vi "TimingDebug.vi"() -> ()   [LabVIEW 2021]
uses:
  <vilib>/DAQmx/read.llb/DAQmx Read (Analog 2D DBL NChan NSamp).vi
  <vilib>/DAQmx/create/channels.llb/DAQmx Create Channel (AI-Voltage-Basic).vi
  <vilib>/DAQmx/configure/timing.llb/DAQmx Timing (Sample Clock).vi
  <vilib>/DAQmx/miscellaneous.llb/DAQmx Fill In Error Info.vi
panel:
  out "data":dbl[][](array[numeric]) format="%0.2f"
  out "Time has Elapsed":bool
  out "Elapsed Time (s)":dbl
  out "Inside Loop":bool
  in  "Inside Loop":dbl
  out "Outside loop":bool
  in  "Outside loop":dbl
  in  "Run Duration (s)":u32=100 caption="Duration (s)"
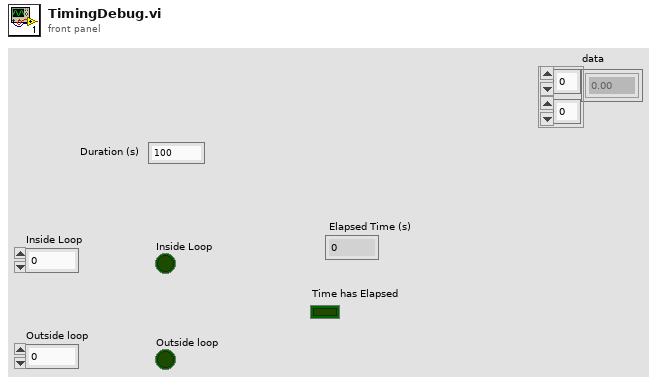
[diagram p1: front panel]
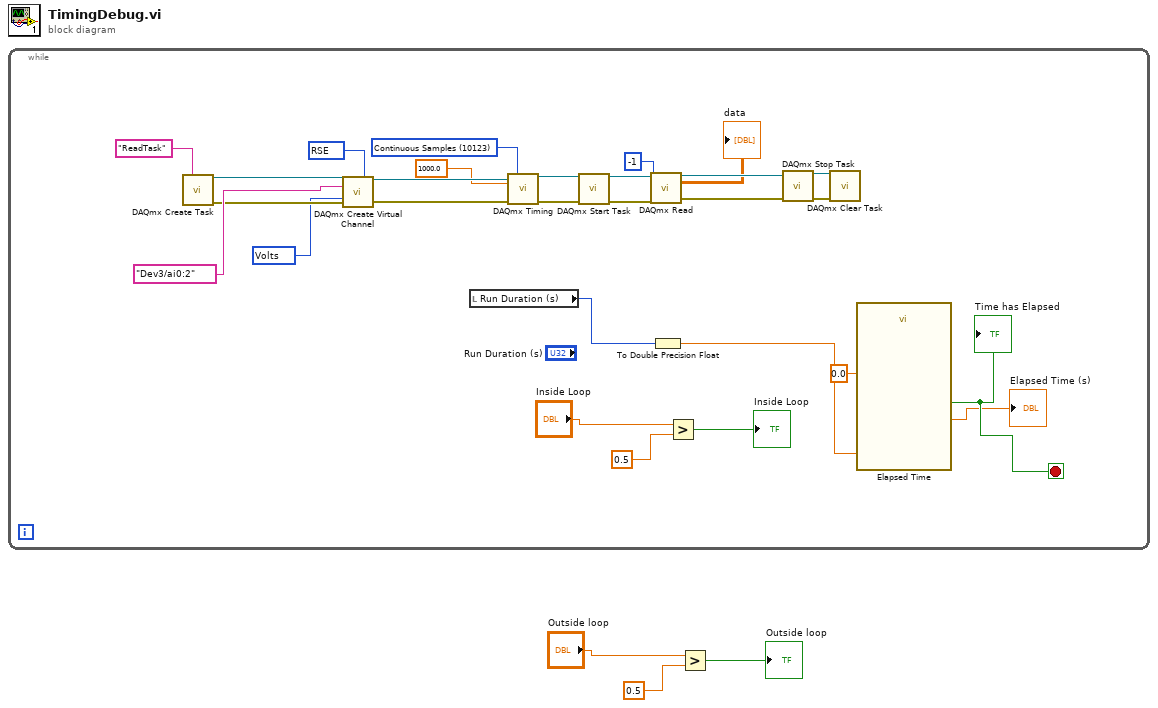
[diagram p0: block diagram]
diagram:
  n1 = while {
    stop <- w27 stop-if-true
    w11 = 10123 items=["Finite Samples"=10178, "Continuous Samples"=10123, "Hardware Timed Single Point"=12522] ("sample mode")
    w12 = 10083 items=["Default"=-1, "RSE"=10083, "NRSE"=10078, "Differential"=10106, "Pseudodifferential"=12529] ("input terminal configuration")
    w13 = 10348 items=["Volts"=10348, "From Custom Scale"=10065] ("units")
    n2 = call <vilib>:"DAQmx Create Task.vi"("new task name"="ReadTask") -> ("task out"=w22:refnum<k21>, "error out"=w15:errorcluster)  [unwired: 13 in]
    n3 = call-poly <vilib>:"DAQmx Create Virtual Channel.vi"("task in"=w22, "input terminal configuration"=w12, "physical channels"=tag "Dev3/ai0:2" ("DAQmx Physical Channel"), "units"=w13, "error in"=w15) -> ("task out"=w21:refnum<k21>, "error out"=w16:errorcluster)  [unwired: 9 in]
    n4 = local read "Run Duration (s)"() -> (w25:u32)
    n5 = call-poly <vilib>:"DAQmx Timing.vi"("task/channels in"=w21, "sample mode"=w11, "rate"=1000.0, "error in"=w16) -> ("task out"=w8:refnum<k21>, "error out"=w5:errorcluster)  [unwired: 10 in]
    n6 = call <vilib>:"DAQmx Start Task.vi"("task/channels in"=w8, "error in"=w5) -> ("task out"=w7:refnum<k21>, "error out"=w6:errorcluster)  [unwired: 12 in]
    n7 = call-poly <vilib>:"DAQmx Read.vi"("task/channels in"=w7, "number of samples per channel"=-1, "error in"=w6) -> ("task out"=w20:refnum<k21>, "data"=→"data":dbl[][], "error out"=w17:errorcluster)  [unwired: 10 in]
    n8 = To Double Precision Float(number=w25) -> (double precision float=w31:dbl)
    n9 = Greater?(x="Inside Loop", y=0.5) -> (0:→"Inside Loop":bool)
    n10 = call <vilib>:"DAQmx Stop Task.vi"("task/channels in"=w20, "error in"=w17) -> ("task out"=w19:refnum<k21>, "error out"=w18:errorcluster)  [unwired: 12 in]
    n11 = call <vilib>:"DAQmx Clear Task.vi"("task in"=w19, "error in"=w18) -> ()  [unwired: 13 in, 1 out]
    n12 = call "Elapsed Time"("Time Target (s)"=w31, "Set Start Time (s)"=0.0) -> ("Elapsed Time (s)"=→"Elapsed Time (s)":dbl, "Time has Elapsed"=w27:bool)  [unwired: 10 in, 6 out]
    "Time has Elapsed" <- w27
  }
  n13 = Greater?(x="Outside loop", y=0.5) -> (0:→"Outside loop":bool)
